vi "Compute Laplacian 64f.vi"(8 "Error In":errorcluster, 10 "Input":T1 {"Dimension"."Width" min=1; "Dimension"."Height" min=1; "Dimension"."Depth" min=1}, 11 "Laplacian Object":T6 {"Laplacian Out"."Dimension"."Width" min=1; "Laplacian Out"."Dimension"."Height" min=1; "Laplacian Out"."Dimension"."Depth" min=1}) -> (0 "Error Out":errorcluster, 3 "Laplacian Out":T1 {"Dimension"."Width" min=1; "Dimension"."Height" min=1; "Dimension"."Depth" min=1}, 4 "Time in ms":dbl)   [LabVIEW 2012, in "OpenCLV x64.lvlib"]
doc: "Computes the Laplacian based on already created Laplacian Object. The dimensions of the input array <b>must</b> match the size of the dimension used to define the Laplacian Object."
uses:
  OpenCLV x64.lvlib
  Controls/Laplacian Object.ctl
  Controls/Device ID.ctl
  Controls/Program Handle.ctl
  Controls/Memory Object.ctl
  Controls/Memory ID.ctl
  User Controls/Array Dimensions.ctl
  Controls/Memory Type.ctl
  Error Checking/Add Error Functional Global.vi
  Set Kernel Arguments/Set Kernel Arguments Memory Object.vi
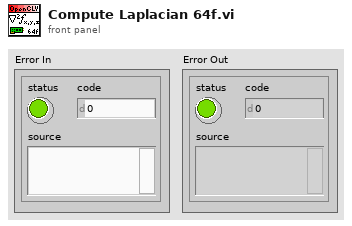
[diagram p1: front panel]
types:
  T1 = typedef "OpenCLV x64.lvlib/Memory Object.ctl" = cluster{"Device ID":T2, "Memeroy ID":T3, "Dimension":T4, "Memory Type":T5}
  T2 = typedef "OpenCLV x64.lvlib/Device ID.ctl" = u64
  T3 = typedef "OpenCLV x64.lvlib/Memory ID.ctl" = u64
  T4 = typedef "Array Dimensions.ctl" = cluster{"Depth":u64, "Height":u64, "Width":u64}
  T5 = typedef "OpenCLV x64.lvlib/Memory Type.ctl" = enum16{"32f", "u8", "i8", "u16", "i16", "u32", "i32", "64f"}
  T6 = typedef "OpenCLV x64.lvlib/Laplacian Object.ctl" = cluster{"Device Out":T2, "Program Handle":T7, "Laplacian Out":T1}
  T7 = typedef "OpenCLV x64.lvlib/Program Handle.ctl" = u64
  T8 = typedef "OpenCLV x64.lvlib/Kernel Handle.ctl" = u64
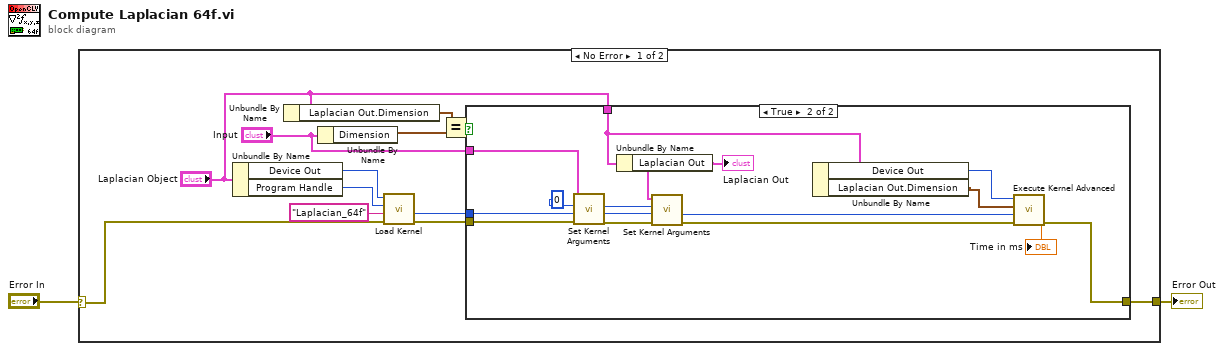
[diagram p0: block diagram]
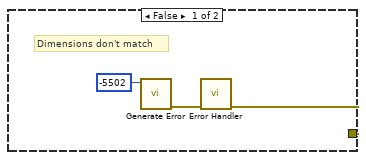
[diagram p2: hidden frame]
diagram:
  n1 = case shown="No Error" "Error In" {
    selector: "Error In" -> [w14 w33]
    tunnel: [w8 w33] -> w1
    frame No Error {
      n2 = Unbundle By Name("Laplacian Object") -> ("Device Out"=w12:T2, "Program Handle"=w13:T7)
      n3 = Unbundle By Name("Laplacian Object") -> ("Laplacian Out.Dimension"=w6:T4)
      n4 = Unbundle By Name("Input") -> ("Dimension"=w5:T4)
      n5 = call "Load Kernel.vi"("Error In"=w14, "Kernel Name"="Laplacian_64f", "Program Handle"=w13, "Device In"=w12) -> ("Error Out"=w10:errorcluster, "Kernel Handle"=w9:T8)  [unwired: 4 in, 2 out]
      n6 = Equal?(x=w6, y=w5) -> (x = y?=w4:bool)
      n7 = case shown="True" w4 {
        tunnel: w10 -> [_ w32]
        tunnel: w9 -> [_ w31]
        tunnel: [w15 w20] -> w8
        tunnel: "Laplacian Object" -> [_ w24]
        tunnel: "Input" -> [_ w23]
        frame False {
          # "Dimensions don't match"
          n8 = call "Generate Error.vi"("Error"=-5502) -> ("error out"=w16:errorcluster)  [unwired: 10 in]
          n9 = call-poly "Error Handler.vi"("Error In"=w16) -> ("Error Out"=w15:errorcluster)  [unwired: 10 in]
        }
        frame True {
          n10 = call-poly "Set Kernel Arguments.vi"("Error In"=w32, "Kernel Handle"=w31, "Argument Number"=0, "Memory Object"=w23) -> ("Error Out"=w27:errorcluster, "Kernel Handle out"=w28:T8, "Auto Inc Arugment Number"=w29:i32)  [unwired: 5 in]
          n11 = Unbundle By Name(w24) -> ("Laplacian Out"=w18:T1)
          "Laplacian Out" <- w18
          n12 = call-poly "Set Kernel Arguments.vi"("Error In"=w27, "Kernel Handle"=w28, "Argument Number"=w29, "Memory Object"=w18) -> ("Error Out"=w21:errorcluster, "Kernel Handle out"=w22:T8)  [unwired: 5 in, 1 out]
          n13 = Unbundle By Name(w24) -> ("Device Out"=w26:T2, "Laplacian Out.Dimension"=w19:T4)
          n14 = call "Execute Kernel Advanced.vi"("Error In"=w21, "Kernel Handle"=w22, "Thread Dimensions"=w19, "Device In"=w26) -> ("Error Out"=w20:errorcluster, "Time in ms"=→"Time in ms":dbl)  [unwired: 4 in, 2 out]
        }
      }
    }
    frame Error {
    }
  }
  "Error Out" <- w1
